vi "OpenDevice.vi"(8 "错误输入（无错误）":errorcluster, 9 "DevIndex":u32, 11 "设备类型":u32(ring)=3 items=["PCI5121"=1, "PCI9810"=2, "USBCAN1"=3, "USBCAN2"=4, "PCI9820"=5, "PCI5110"=7, "PC104CAN"=11, "CANETUDP"=12, "PCI9840B"=14, "PC104C2"=15, "PCI9820I"=16, "CANETTCP"=17, "PCIE9221"=24, "PCI5010U"=19, "USBCAN_E_U"=20, "USBCAN_2E_U"=21, "PCI5020U"=22]) -> (0 "错误输出":errorcluster, 1 "DevInd":u32, 2 "Result":bool, 3 "DevType":u32)   [LabVIEW 2013]
uses:
  ControlCAN.dll
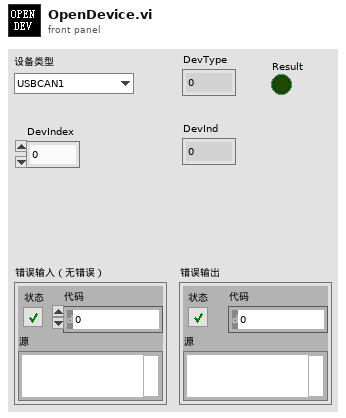
[diagram p1: front panel]
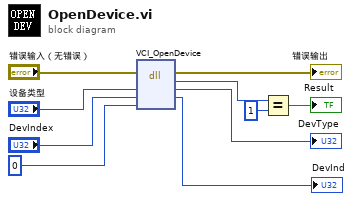
[diagram p0: block diagram]
diagram:
  n1 = dll-call lib="PTH1`abs E桌面休眠电流方案休眠电流源码20181130\nInstrumentCANControlCAN.dll" fn="VCI_OpenDevice"(error in="错误输入（无错误）", "DevType"="设备类型", "DevIndex"="DevIndex", "Reserved"=u32 0) -> (error out=→"错误输出":errorcluster, "返回类型"=w10:u32, "DevType"=→"DevType":u32, "DevIndex"=→"DevInd":u32)  [unwired: 3 in, 1 out]
  n2 = Equal?(x=w10, y=u32 1) -> (x = y?=→"Result":bool)
